vi "Interpolate 2D Scattered.vi"   [LabVIEW 2020, in "NI_AAL_Interpolation.lvlib"]
doc: "Performs two-dimensional interpolation on scattered points."
uses:
  <vilib>/gmath/NI_AAL_Interpolation.lvlib
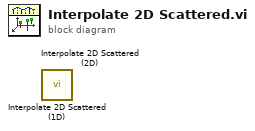
[diagram p0: block diagram]
diagram:
  n1 = call <vilib>:"Interpolate 2D Scattered (1D).vi"() -> ()  [unwired: 10 in, 2 out]
  n2 = call <vilib>:"Interpolate 2D Scattered (2D).vi"() -> ()  [unwired: 10 in, 2 out]
